vi "Periodic Tasks.vi"() -> ()   [LabVIEW 2011]
doc: "This VI runs in parallel to other tasks. It can contain as many user-defined periodic loops as you need. These can carry out PID or other sorts of timed response."
uses:
  <vilib>/Platform/TimedLoop/XDataNode/timing_clust.ctl
  <vilib>/Platform/TimedLoop/XDataNode/nitl_modes.ctl
  <vilib>/Platform/TimedLoop/XDataNode/wakeup.ctl
  <vilib>/Rock Robotics/SystemInterfaces/Utilities/FPGA_UtilitiesLED State.ctl
  <vilib>/Rock Robotics/SystemInterfaces/Utilities/FPGA_UtilitiesLED Source.ctl
  <vilib>/Rock Robotics/WPI/Relay/WPI_RelayValue.ctl
  Robot Global Data.vi
  <vilib>/Platform/TimedLoop/XDataNode/XDataNode.xnode
  <vilib>/Platform/TimedLoop/XDataNode/XDNodeRunTimeDep.lvlib
panel:
  in  "Enable Home":bool
  in  "Home Speed":dbl
  in  "Home Position":dbl
  out "Current Voltage":dbl
  in  "upper limit":dbl=4.5
  in  "lower limit":dbl=0.85
  # "Speed to move to home"
  # "Target Tracking"
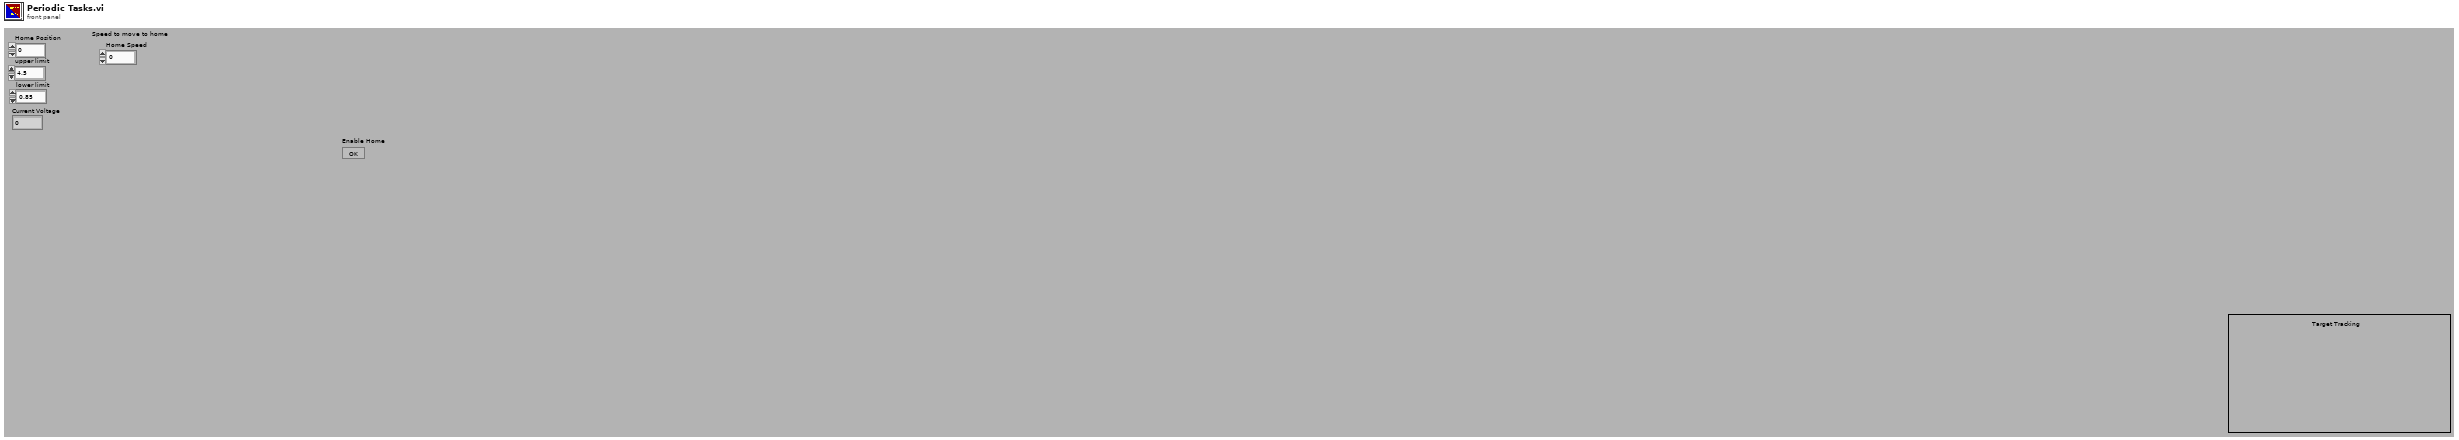
[diagram p1: front panel]
types:
  T1 = typedef "XDNodeRunTimeDep.lvlib/timing_clust.ctl" = cluster{"Expected End [f-1]":u64, "Actual End [f-1]":u64, "Finished Late? [f-1]":bool, "Expected End [i-1]":u64, "Actual End [i-1]":u64, "Finished Late? [i-1]":bool, "Expected Start [i]":u64, "Actual Start [i]":u64, "Expected Start [f]":u64, "Actual Start [f]":u64, "Source Name":string, "Structure Name":string, "Period":i64, "Deadline":i64, "Offset":i64, "Start":i64, "Priority":i32, "Timeout":i32, "Mode":T2, "Wakeup Reason":T3, "Error":errorcluster, "Source Type":string, "Secondary Source Type":string, "Global End Time":u64, "Global Start Time":u64, "Frame Duration":u64, "Iteration Duration":u64, "Assigned CPU":i32, "I/O Scan Engine Mode":u32}
  T2 = typedef "XDNodeRunTimeDep.lvlib/nitl_modes.ctl" = enum32{"No Change", "Process missed periods, maintain original phase", "Discard missed periods, maintain original phase", "Process missed periods, ignore original phase", "Discard missed periods, ignore original phase"}
  T3 = typedef "XDNodeRunTimeDep.lvlib/wakeup.ctl" = enum32{"Normal", "Aborted", "Asynchronous wakeup", "Timing source error", "Timed loop error", "Timeout"}
  T4 = typedef "WPI_RelayValue.ctl" = enum16{"Off", "On", "Forward", "Reverse"}
  T5 = typedef "WPI_AnalogChannelDevRef.ctl" = cluster{"DevStatus":errorcluster, "Analog Module":T6, "Analog Channel":T7}
  T6 = typedef "FPGA_TypedefAnalogModule.ctl" = enum16{"Analog Module 1", "Analog Module 2"}
  T7 = typedef "FPGA_AIChannel.ctl" = enum8{"AI 1", "AI 2", "AI 3", "AI 4", "AI 5", "AI 6", "AI 7", "AI 8", "Invalid"}
  T8 = typedef "WPI_RelayDevRef.ctl" = cluster{"DevStatus":errorcluster, "Relay Channel":T9, "Digital Module":T10, "Relay Direction":T11}
  T9 = typedef "FPGA_DIORelayChannel.ctl" = enum8{"Relay 1", "Relay 2", "Relay 3", "Relay 4", "Relay 5", "Relay 6", "Relay 7", "Relay 8", "Invalid"}
  T10 = typedef "FPGA_TypedefDigitalModule.ctl" = enum16{"Digital Module 1", "Digital Module 2"}
  T11 = typedef "WPI_RelayDirection.ctl" = enum16{"Both directions", "Forward only", "Reverse only"}
  T12 = cluster{"Axis 1":dbl, "Axis 2":dbl, "Axis 3":dbl, "Axis 4":dbl, "Axis 5":dbl, "Axis 6":dbl, "Button 1":bool, "Button 2":bool, "Button 3":bool, "Button 4":bool, "Button 5":bool, "Button 6":bool, "Button 7":bool, "Button 8":bool, "Button 9":bool, "Button 10":bool, "Button 11":bool, "Button 12":bool}
  T13 = cluster{"Driver Station Digital Output (1-8)[0]":bool, "Driver Station Digital Output (1-8)[1]":bool, "Driver Station Digital Output (1-8)[2]":bool, "Driver Station Digital Output (1-8)[3]":bool, "Driver Station Digital Output (1-8)[4]":bool, "Driver Station Digital Output (1-8)[5]":bool, "Driver Station Digital Output (1-8)[6]":bool, "Driver Station Digital Output (1-8)[7]":bool, "Driver Station Digital Output (1-8)[8]":bool}
  T14 = typedef "FPGA_UtilitiesLED State.ctl" = enum16{"Off", "On", "Toggle"}
  T15 = typedef "FPGA_UtilitiesLED Source.ctl" = enum16{"User LED", "FPGA LED"}
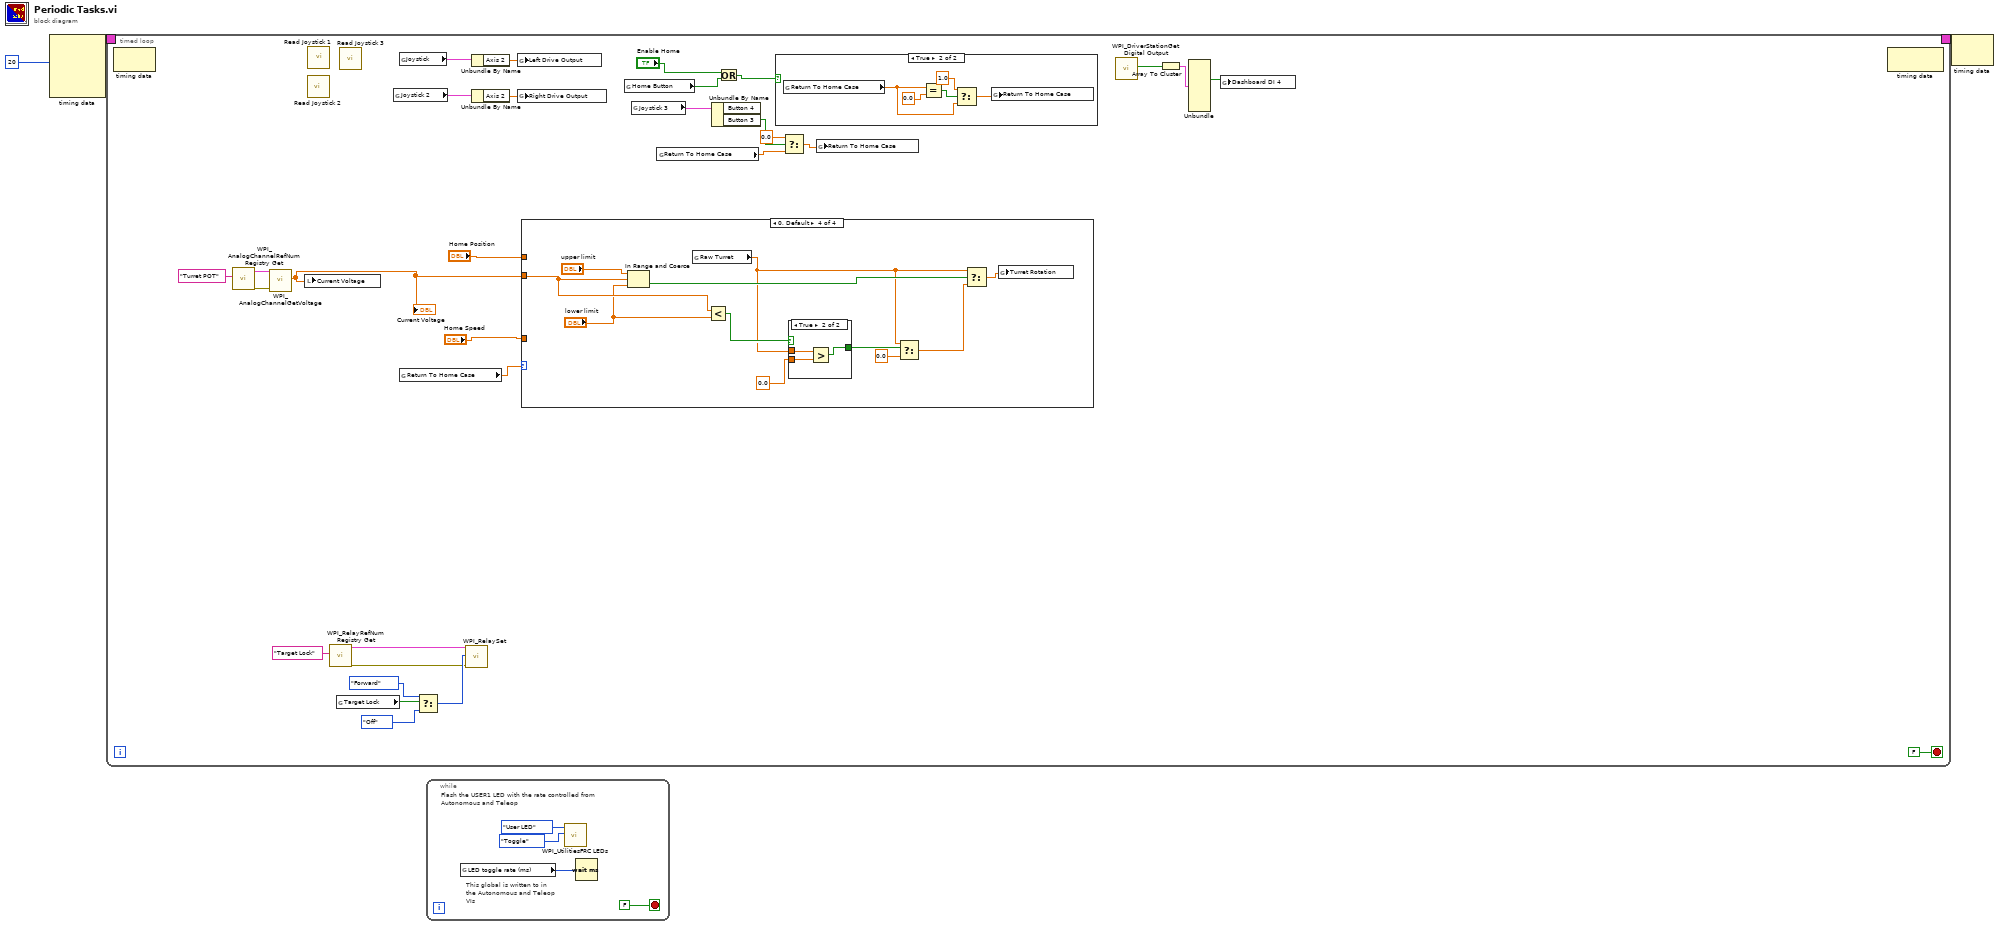
[diagram p0: block diagram]
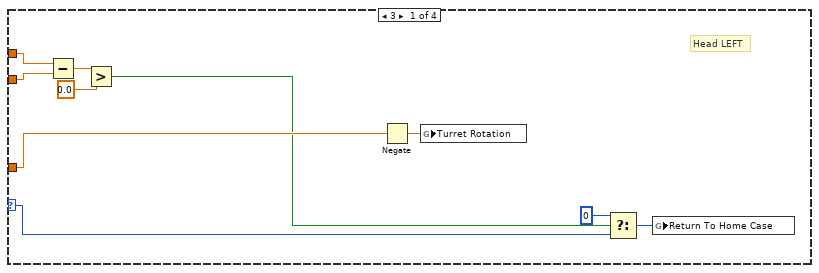
[diagram p2: hidden frame]
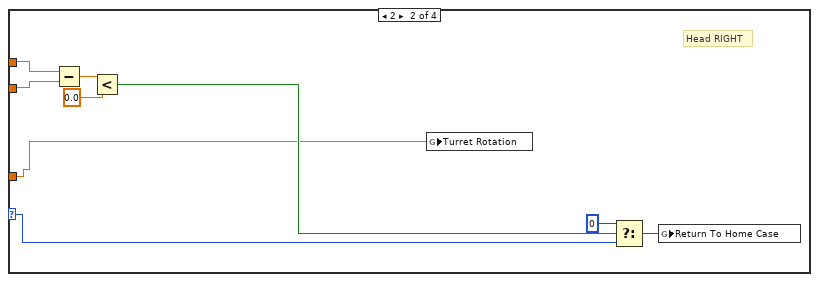
[diagram p3: hidden frame]
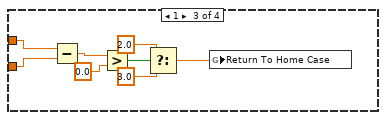
[diagram p4: hidden frame]
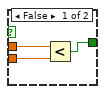
[diagram p5: hidden frame]
diagram:
  n1 = node-c288(i64 20 ("Period")) -> (w3:T1)  [unwired: 3 in]
  n2 = timed-loop {
    timing: w3 -> [_]
    timing-out: [_] -> w2
    stop <- FALSE stop-if-true
    n3 = node-c288() -> ()  [unwired: 1 in, 1 out]
    n4 = call <vilib>:"WPI_AnalogChannelRefNum Registry Get.vi"("refnum name"="Turret POT") -> ("error out"=w17:errorcluster, "AIDeviceRef"=w18:T5)  [unwired: 9 in]
    n5 = call <vilib>:"WPI_AnalogChannelGetVoltage.vi"("error in (no error)"=w17, "AIDeviceRef"=w18) -> ("Voltage"=w14:dbl)  [unwired: 7 in, 2 out]
    "Current Voltage" <- w14
    n6 = local write "Current Voltage"(w14) -> ()
    n7 = call "Read Joystick 2.vi"() -> ()  [unwired: 12 in]
    n8 = call "Read Joystick 1.vi"() -> ()  [unwired: 12 in]
    n9 = call <vilib>:"WPI_RelayRefNum Registry Get.vi"("refnum name"="Target Lock") -> ("error out"=w19:errorcluster, "RelayDevRef"=w20:T8)  [unwired: 9 in]
    n10 = global read "Robot Global Data.vi" "Target Lock"() -> (w25:bool)
    n11 = call "Read Joystick 3.vi"() -> ()  [unwired: 12 in]
    n12 = global read "Robot Global Data.vi" "Joystick 2"() -> (w27:T12)
    n13 = global read "Robot Global Data.vi" "Joystick"() -> (w28:T12)
    n14 = global read "Robot Global Data.vi" "Return To Home Case"() -> (w13:dbl)
    n15 = Select(t=WPI_RelayValue."Forward" ("RelayValue"), s=w25, f=WPI_RelayValue."Off" ("RelayValue")) -> (s? t:f=w22:T4)
    n16 = call <vilib>:"WPI_RelaySet.vi"("error in (no error)"=w19, "RelayValue"=w22, "RelayDevRef"=w20) -> ()  [unwired: 7 in, 2 out]
    n17 = Unbundle By Name(w28) -> ("Axis 2"=w30:dbl)
    n18 = Unbundle By Name(w27) -> ("Axis 2"=w29:dbl)
    n19 = global write "Robot Global Data.vi" "Left Drive Output"(w30) -> ()
    n20 = global write "Robot Global Data.vi" "Right Drive Output"(w29) -> ()
    n21 = case shown="0, Default" w13 {
      selector: w13 -> [w41 w45 _ _]
      tunnel: w14 -> [w37 w46 w59 w71]
      tunnel: "Home Position" -> [w38 w47 w60 _]
      tunnel: "Home Speed" -> [w39 w44 _ _]
      frame 3 {
        # "Head LEFT"
        n22 = Subtract(x=w38, y=w37) -> (x-y=w36:dbl)
        n23 = Greater?(x=w36, y=0.0) -> (0:w34:bool)
        n24 = Negate(x=w39) -> (-x=w40:dbl)
        n25 = global write "Robot Global Data.vi" "Turret Rotation"(w40) -> ()
        n26 = Select(t=0, s=w34, f=w41) -> (s? t:f=w42:i32)
        n27 = global write "Robot Global Data.vi" "Return To Home Case"(w42) -> ()
      }
      frame 2 {
        # "Head RIGHT"
        n28 = Subtract(x=w47, y=w46) -> (x-y=w50:dbl)
        n29 = Less?(x=w50, y=0.0) -> (x < y?=w48:bool)
        n30 = global write "Robot Global Data.vi" "Turret Rotation"(w44) -> ()
        n31 = Select(t=0, s=w48, f=w45) -> (s? t:f=w51:i32)
        n32 = global write "Robot Global Data.vi" "Return To Home Case"(w51) -> ()
      }
      frame 1 {
        n33 = Subtract(x=w60, y=w59) -> (x-y=w58:dbl)
        n34 = Greater?(x=w58, y=0.0) -> (0:w56:bool)
        n35 = Select(t=2.0, s=w56, f=3.0) -> (s? t:f=w53:dbl)
        n36 = global write "Robot Global Data.vi" "Return To Home Case"(w53) -> ()
      }
      frame 0, Default {
        n37 = In Range and Coerce(upper limit="upper limit", x=w71, lower limit="lower limit") -> (In Range?=w68:bool)  [unwired: 1 out]
        n38 = global read "Robot Global Data.vi" "Raw Turret"() -> (w61:dbl)
        n39 = Less?(x=w71, y="lower limit") -> (x < y?=w63:bool)
        n40 = case shown="True" w63 {
          tunnel: 0.0 -> [w73 w77]
          tunnel: [w72 w76] -> w64
          tunnel: w61 -> [w74 w75]
          frame False {
            n41 = Less?(x=w74, y=w73) -> (x < y?=w72:bool)
          }
          frame True {
            n42 = Greater?(x=w75, y=w77) -> (0:w76:bool)
          }
        }
        n43 = Select(t=w61, s=w64, f=0.0) -> (s? t:f=w62:dbl)
        n44 = Select(t=w61, s=w68, f=w62) -> (s? t:f=w70:dbl)
        n45 = global write "Robot Global Data.vi" "Turret Rotation"(w70) -> ()
      }
    }
    n46 = global read "Robot Global Data.vi" "Home Button"() -> (w5:bool)
    n47 = global read "Robot Global Data.vi" "Joystick 3"() -> (w26:T12)
    n48 = global read "Robot Global Data.vi" "Return To Home Case"() -> (w10:dbl)
    n49 = Unbundle By Name(w26) -> ("Button 3"=w11:bool)  [unwired: 1 out]
    n50 = Or(x="Enable Home", y=w5) -> (x .or. y?=w4:bool)
    n51 = case shown="True" w4 {
      frame False {
      }
      frame True {
        n52 = global read "Robot Global Data.vi" "Return To Home Case"() -> (w79:dbl)
        n53 = Equal?(x=w79, y=0.0) -> (x = y?=w81:bool)
        n54 = Select(t=1.0, s=w81, f=w79) -> (s? t:f=w78:dbl)
        n55 = global write "Robot Global Data.vi" "Return To Home Case"(w78) -> ()
      }
    }
    n56 = Select(t=0.0, s=w11, f=w10) -> (s? t:f=w9:dbl)
    n57 = global write "Robot Global Data.vi" "Return To Home Case"(w9) -> ()
    n58 = call <vilib>:"WPI_DriverStationGet Digital Output.vi"() -> ("Driver Station Digital Output (1-8)"=w33:bool[])  [unwired: 10 in, 1 out]
    n59 = Array To Cluster(array=w33) -> (cluster=w32:T13)
    n60 = Unbundle(w32) -> ("Driver Station Digital Output (1-8)[3]"=w31:bool)  [unwired: 8 out]
    n61 = global write "Robot Global Data.vi" "Dashboard DI 4"(w31) -> ()
    n62 = node-c288() -> ()  [unwired: 1 in, 1 out]
  }
  n63 = while {
    stop <- FALSE stop-if-true
    # "This global is written to in the Autonomous and Teleop VIs"
    # "Flash the USER1 LED with the rate controlled from Autonomous and Teleop"
    n64 = global read "Robot Global Data.vi" "LED toggle rate (ms)"() -> (w85:u32)
    n65 = call <vilib>:"WPI_UtilitiesFRC LEDs.vi"("State"=FPGA_UtilitiesLED_State."Toggle", "LED Type"=FPGA_UtilitiesLED_Source."User LED") -> ()  [unwired: 1 in, 9 out]
    n66 = Wait (ms)(milliseconds to wait=w85) -> ()  [unwired: 1 out]
  }
  n67 = node-c288(w2) -> ()  [unwired: 1 out]
